vi "WSVCAP SHL Host LL I2C Semaphore Global.vi"() -> ()   [LabVIEW 2017]
panel:
  in  "Ctl Mgr Semaphores":T1[](array[typedef])
  in  "IF Core Semaphores":T1[](array[typedef])
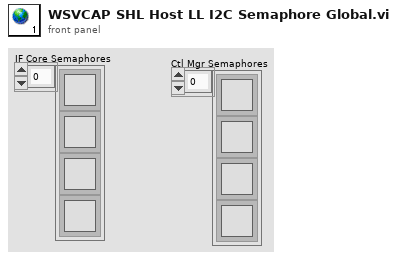
[diagram p1: front panel]
types:
  T1 = typedef "Semaphore RefNum" = refnum<k1>
diagram:
